vi "LLB Pre-Build CHM Build.vi"(6 "Top Level/Always Included VIs":path[](array[path]), 7 "Main Destination Path":path, 9 "Target Name":string, 10 "Build Specification Name":string, 11 "Project Path":path) -> (0 "error out":errorcluster)   [LabVIEW 2016]
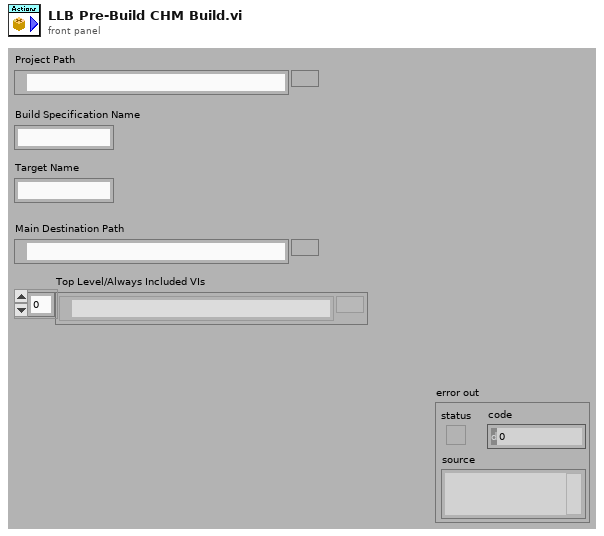
[diagram p1: front panel]
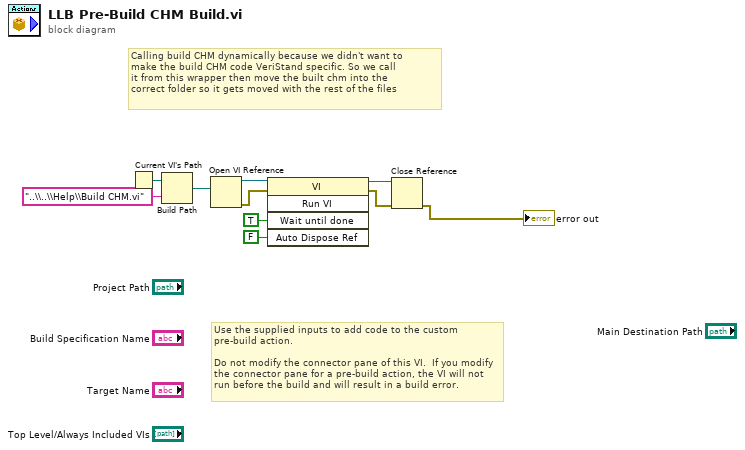
[diagram p0: block diagram]
diagram:
  # "Calling build CHM dynamically because we didn't want to \nmake the build CHM code VeriStand specific. So we call\nit from this wrapper then move the built chm into the\ncorrect folder so it gets moved with the rest of the files"
  # "Use the supplied inputs to add code to the custom pre-build action.\n\nDo not modify the connector pane of this VI.  If you modify the connector pane for a pre-build action, the VI will not run before the build and will result in a build error."
  n1 = Current VI's Path() -> (path=w10:path)
  n2 = Build Path(base path=w10, name or relative path="..\\..\\Help\\Build CHM.vi") -> (appended path=w2:path)
  n3 = Open VI Reference(vi path=w2) -> (vi reference=w8:refnum<vi>, error out=w7:errorcluster)  [unwired: 5 in]
  n4 = invoke class="VI" method="Run VI"(reference=w8, error in=w7, "Wait until done"=TRUE ("Wait Until Done"), "Auto Dispose Ref"=FALSE ("Auto Dispose Reference")) -> (reference out=w4:refnum<vi>, error out=w3:errorcluster)  [unwired: 1 in, 3 out]
  n5 = Close Reference(reference=w4, error in (no error)=w3) -> (error out=→"error out":errorcluster)
